vi "svl_Check Highpass Cutoff Frequency.vi"(6 "highpass cutoff frequency":dbl=1.0 format="%.2f", 7 "reset (in)":bool, 8 "error in (no error)":errorcluster) -> (0 "error out":errorcluster, 2 "parameter has changed":bool)   [LabVIEW 2017, in "SoundVib_Integration.lvlib"]
uses:
  <vilib>/addons/Sound and Vibration/svt_Integration/SoundVib_Integration.lvlib
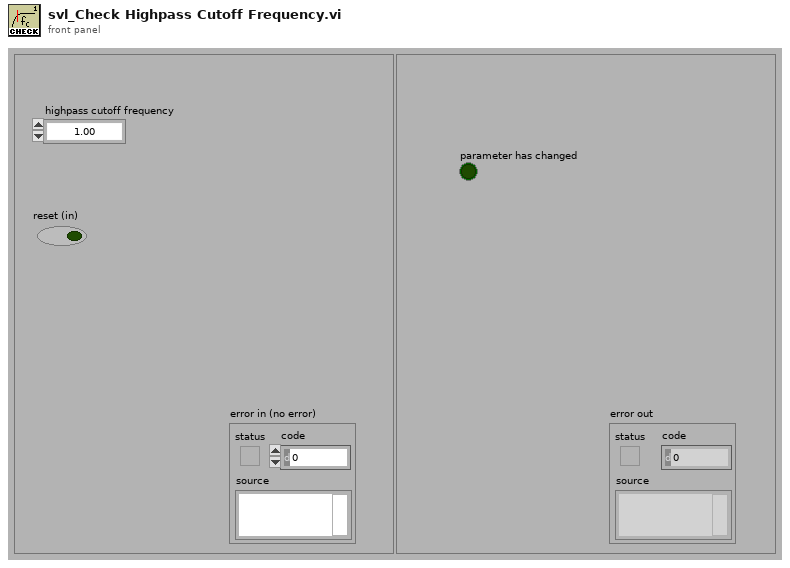
[diagram p1: front panel]
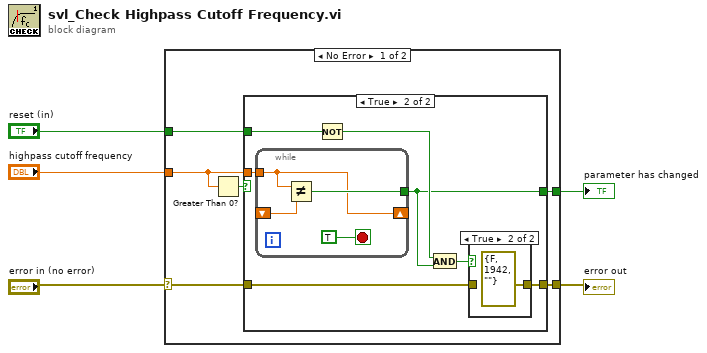
[diagram p0: block diagram]
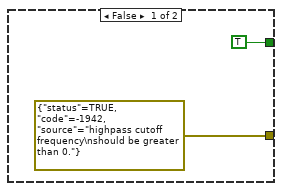
[diagram p2: hidden frame]
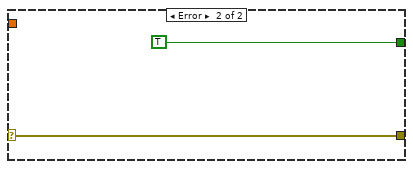
[diagram p4: hidden frame]
diagram:
  n1 = case shown="No Error" "error in (no error)" {
    selector: "error in (no error)" -> [w10 w28]
    tunnel: [w8 TRUE] -> w5
    tunnel: [w9 w28] -> w3
    tunnel: "highpass cutoff frequency" -> [w7 _]
    tunnel: "reset (in)" -> [w6 _]
    frame No Error {
      n2 = Greater Than 0?(x=w7) -> (x > 0?=w11:bool)
      n3 = case shown="True" w11 {
        tunnel: w10 -> [_ w20]
        tunnel: [errorcluster {"status"=TRUE, "code"=-1942, "source"="highpass cutoff frequency\nshould be greater than 0."} ("error IO") w19] -> w9
        tunnel: [TRUE w14] -> w8
        tunnel: w7 -> [_ w18]
        tunnel: w6 -> [_ w17]
        frame False {
        }
        frame True {
          n4 = while {
            tunnel: w18 -> [w21]
            tunnel: [w23] -> w14
            shift-left: _ -> [w22]
            shift-right: [w21] -> _
            stop <- TRUE stop-if-true
            n5 = Not Equal?(x=w21, y=w22) -> (x != y?=w23:bool)
          }
          n6 = Not(x=w17) -> (.not. x?=w16:bool)
          n7 = And(x=w16, y=w14) -> (x .and. y?=w15:bool)
          n8 = case shown="True" w15 {
            tunnel: w20 -> [w25 _]
            tunnel: [w25 errorcluster {"status"=FALSE, "code"=1942, "source"=""} ("error IO")] -> w19
            frame False {
            }
            frame True {
            }
          }
        }
      }
    }
    frame Error {
    }
  }
  "error out" <- w3
  "parameter has changed" <- w5
